vi "Pump Status.vi"(8 "error in (no error)":errorcluster, 11 "FLOM Settings In":T1) -> (0 "error out":errorcluster, 1 "Connection Error":bool, 2 "Pump On?":enum16{"Off", "On", "Not Initialized"}(ring), 3 "FLOM Settings Out":T1={"VISA resource name"="", "Simulated?"=TRUE, "Pump Number"=0.0}, 4 "Pressure":dbl, 5 "Flow Rate":dbl)   [LabVIEW 2021, in "FLOM Pump.lvlib"]
uses:
  FLOM Pump.lvlib
  Settings Cluster.ctl
  <vilib>/Instr/_visa.llb/VISA Flush IO Buffer Mask.ctl
  <vilib>/Instr/_visa.llb/VISA Configure Serial Port (Instr).vi
  <vilib>/regexp/Match Regular Expression.xnode
panel:
  out "concatenated string":string
  out "read buffer":string
  out "result string":string
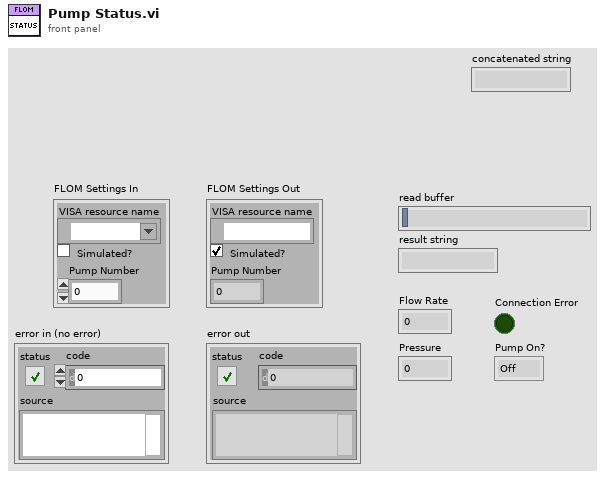
[diagram p1: front panel]
types:
  T1 = typedef "FLOM Pump.lvlib/Settings Cluster.ctl" = cluster{"VISA resource name":refnum<visa-resource-name>, "Simulated?":bool, "Pump Number":dbl}
  T2 = typedef "VISA Flush IO Buffer Mask.ctl" = u16
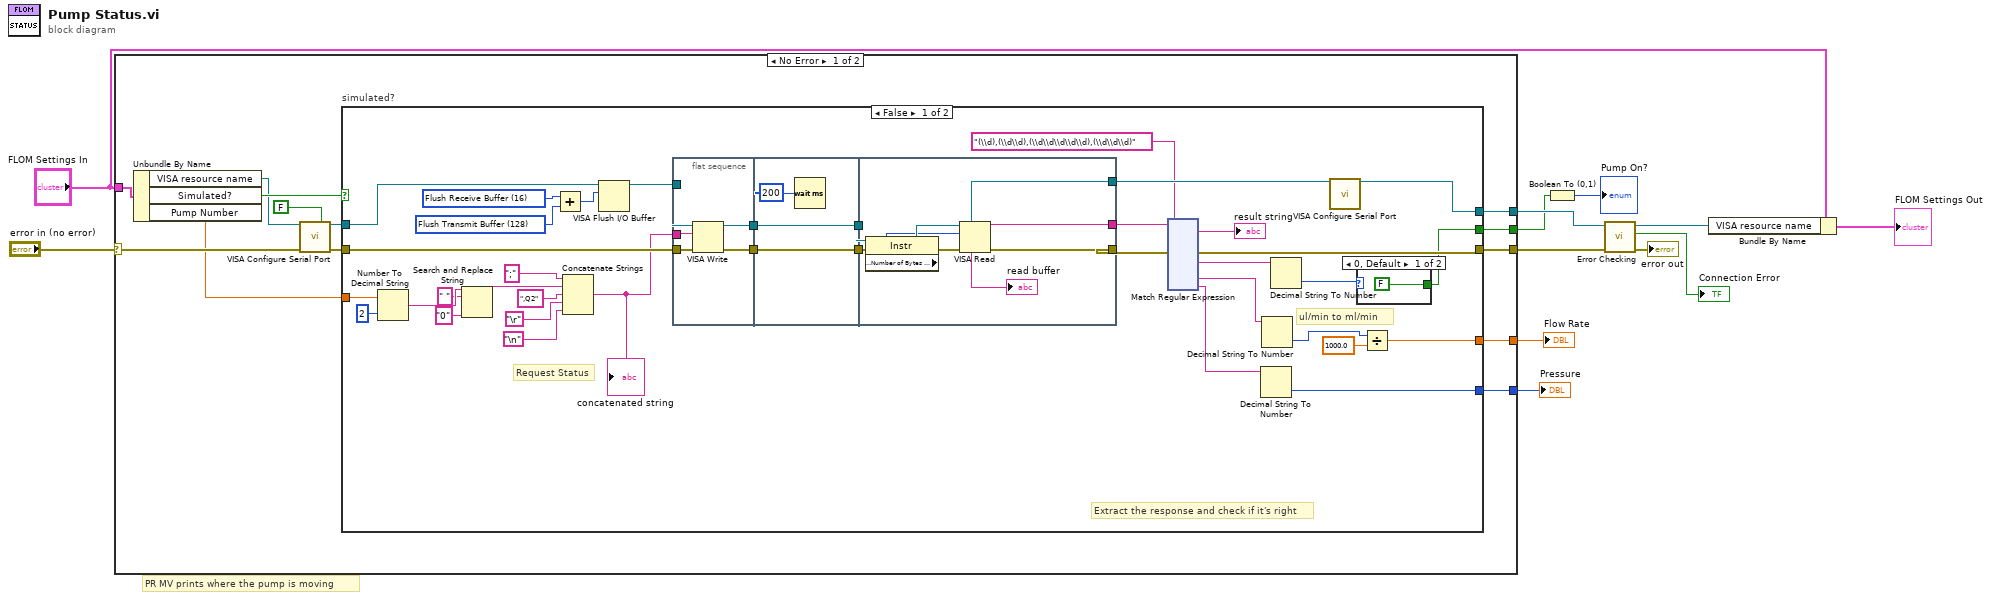
[diagram p0: block diagram]
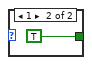
[diagram p2: hidden frame]
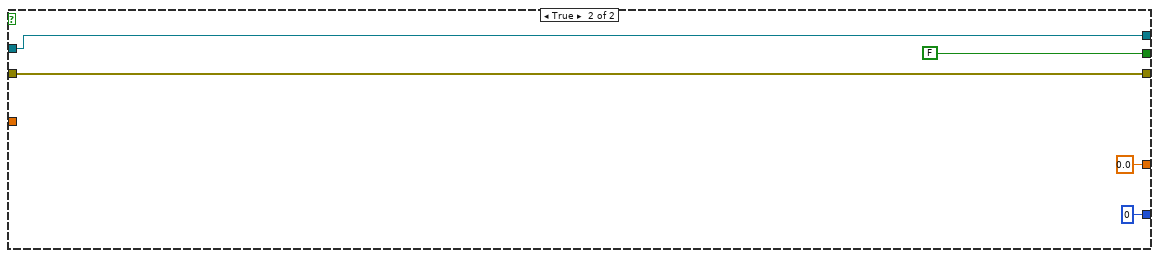
[diagram p3: hidden frame]
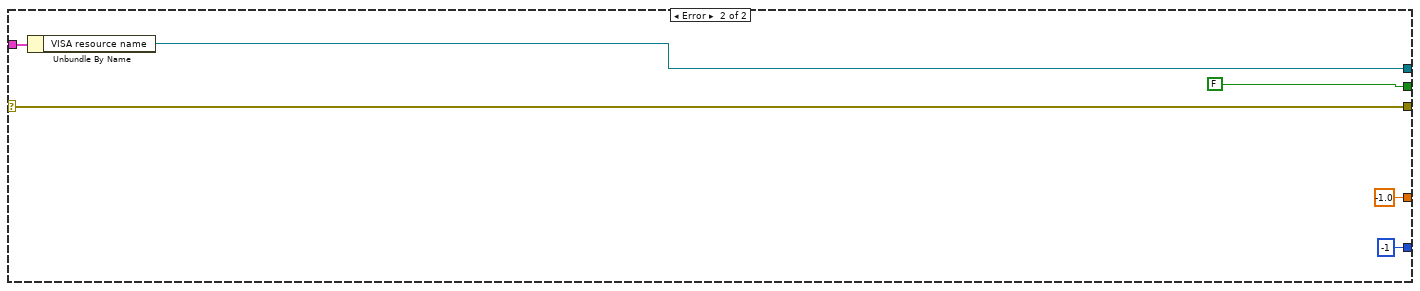
[diagram p4: hidden frame]
diagram:
  # "PR MV prints where the pump is moving"
  n1 = case shown="No Error" "error in (no error)" {
    selector: "error in (no error)" -> [w18 w213]
    tunnel: [w25 w213] -> w10
    tunnel: "FLOM Settings In" -> [w24 w212]
    tunnel: [w23 w211] -> w8
    tunnel: [w16 FALSE] -> w5
    tunnel: [w14 -1.0] -> w2
    tunnel: [w13 -1] -> w1
    frame No Error {
      n2 = Unbundle By Name(w24) -> ("VISA resource name"=w21:refnum<visa-resource-name>, "Simulated?"=w22:bool, "Pump Number"=w15:dbl)
      n3 = call-poly "VISA Configure Serial Port"("VISA resource name"=w21, "Enable Termination\nChar (T)"=FALSE ("Enable Termination\nChar (T)"), "error in (no error)"=w18) -> ("VISA resource name out"=w20:refnum<visa-resource-name>, "error out"=w17:errorcluster)  [unwired: 11 in]
      n4 = case "simulated?" shown="False" w22 {
        tunnel: [w42 w207] -> w25
        tunnel: [w51 w205] -> w23
        tunnel: w17 -> [w62 w207]
        tunnel: w20 -> [w57 w205]
        tunnel: [w39 FALSE] -> w16
        tunnel: w15 -> [w31 _]
        tunnel: [w27 0.0] -> w14
        tunnel: [w26 0] -> w13
        frame False {
          w53 = T2 128 items=["Flush Receive Buffer"=16, "Write Transmit Buffer to Device"=32, "Flush Receive Buffer (No I/O)"=64, "Flush Transmit Buffer"=128] ("Mask")
          w54 = T2 16 items=["Flush Receive Buffer"=16, "Write Transmit Buffer to Device"=32, "Flush Receive Buffer (No I/O)"=64, "Flush Transmit Buffer"=128] ("Mask")
          # "ul/min to ml/min"
          # "Extract the response and check if it's right"
          # "Request Status"
          n5 = Number To Decimal String(number=w31, width (-)=i16 2) -> (decimal integer string=w34:string)
          n6 = Search and Replace String(input string=w34, search string=" ", replace string="0" ("replace string (\"\")")) -> (result string=w30:string)  [unwired: 5 in, 3 out]
          n7 = Add(x=w54, y=w53) -> (x+y=w55:T2)
          n8 = Concatenate Strings(";" ("string"), w30, ",Q2" ("string"), "\r", "\n") -> (w46:string)
          "concatenated string" <- w46
          n9 = VISA Flush I/O Buffer(VISA resource name=w57, mask (16)=w55) -> (VISA resource name out=w56:refnum<visa-resource-name>)  [unwired: 1 in, 1 out]
          n10 = flat-sequence {
            tunnel: [w190] -> w61
            tunnel: [w191] -> w60
            tunnel: w62 -> [w188]
            tunnel: w56 -> [w189]
            tunnel: w46 -> [w187]
            tunnel: w61 -> [w192]
            tunnel: w60 -> [w194]
            tunnel: [w194] -> w59
            tunnel: [w192] -> w58
            tunnel: w59 -> [w202]
            tunnel: w58 -> [w201]
            tunnel: [w197] -> w45
            tunnel: [w196] -> w52
            tunnel: [w195] -> w44
            frame #0 {
              n11 = VISA Write(VISA resource name=w189, write buffer=w187, error in (no error)=w188) -> (VISA resource name out=w190:refnum<visa-resource-name>, error out=w191:errorcluster)  [unwired: 1 out]
            }
            frame #1 {
              n12 = Wait (ms)(milliseconds to wait=u32 200) -> ()  [unwired: 1 out]
            }
            frame #2 {
              n13 = property class="Instr"(reference=w201, error in=w202) -> (reference out=w200:refnum<visa-resource-name>, error out=w199:errorcluster, "Serial Settings:Number of Bytes at Serial Port"=w198:u32)
              n14 = VISA Read(VISA resource name=w200, byte count=w198, error in (no error)=w199) -> (VISA resource name out=w196:refnum<visa-resource-name>, read buffer=w197:string, error out=w195:errorcluster)  [unwired: 1 out]
              "read buffer" <- w197
            }
          }
          n15 = xnode "Match Regular Expression"("input string"=w45, "regular expression"="(\\d),(\\d\\d),(\\d\\d\\d\\d\\d),(\\d\\d\\d)", "error in"=w44) -> ("whole match"=→"result string":string, "error out"=w42:errorcluster, "submatch 1"=w41:string, "submatch 3"=w37:string, "submatch 4"=w36:string)  [unwired: 3 in, 4 out]
          n16 = Decimal String To Number(string=w36) -> (number=w26:i32)  [unwired: 2 in, 1 out]
          n17 = Decimal String To Number(string=w37) -> (number=w28:i32)  [unwired: 2 in, 1 out]
          n18 = Decimal String To Number(string=w41) -> (number=w40:i32)  [unwired: 2 in, 1 out]
          n19 = call-poly "VISA Configure Serial Port"("VISA resource name"=w52) -> ("VISA resource name out"=w51:refnum<visa-resource-name>)  [unwired: 13 in, 1 out]
          n20 = case shown="0, Default" w40 {
            tunnel: [FALSE TRUE] -> w39
            frame 0, Default {
            }
            frame 1 {
            }
          }
          n21 = Divide(x=w28, y=1000.0) -> (x/y=w27:dbl)
        }
        frame True {
        }
      }
    }
    frame Error {
      n22 = Unbundle By Name(w212) -> ("VISA resource name"=w211:refnum<visa-resource-name>)
    }
  }
  "Flow Rate" <- w2
  "Pressure" <- w1
  n23 = Boolean To (0,1)(Boolean=w5) -> (0, 1=→"Pump On?":i16)
  n24 = call "Error Checking.vi"("error in (no error)"=w10, "VISA resource name"=w8) -> ("error out"=→"error out":errorcluster, "Connection Error"=→"Connection Error":bool, "VISA resource name"=w7:refnum<visa-resource-name>)  [unwired: 7 in]
  n25 = Bundle By Name(cluster="FLOM Settings In", "VISA resource name"=w7) -> (→"FLOM Settings Out":T1)
